vi "ReadWriteLoopCase3.vi"() -> ()   [LabVIEW 2019]
uses:
  <vilib>/DAQmx/read.llb/DAQmx Read (Analog DBL 1Chan 1Samp).vi
  <vilib>/DAQmx/write.llb/DAQmx Write (Analog DBL 1Chan 1Samp).vi
  <vilib>/DAQmx/create/channels.llb/DAQmx Create Channel (AI-Voltage-Basic).vi
  <vilib>/DAQmx/configure/timing.llb/DAQmx Timing (Sample Clock).vi
  <vilib>/DAQmx/create/channels.llb/DAQmx Create Channel (AO-Voltage-Basic).vi
  <vilib>/DAQmx/miscellaneous.llb/DAQmx Fill In Error Info.vi
  <resource>/objmgr/daqmx.rc
panel:
  out "error out":errorcluster
  out "Slide":dbl(slide) scale=2900.0..3100.0
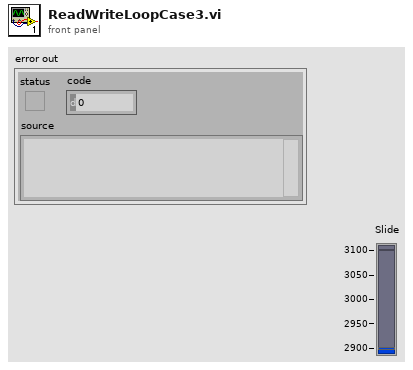
[diagram p1: front panel]
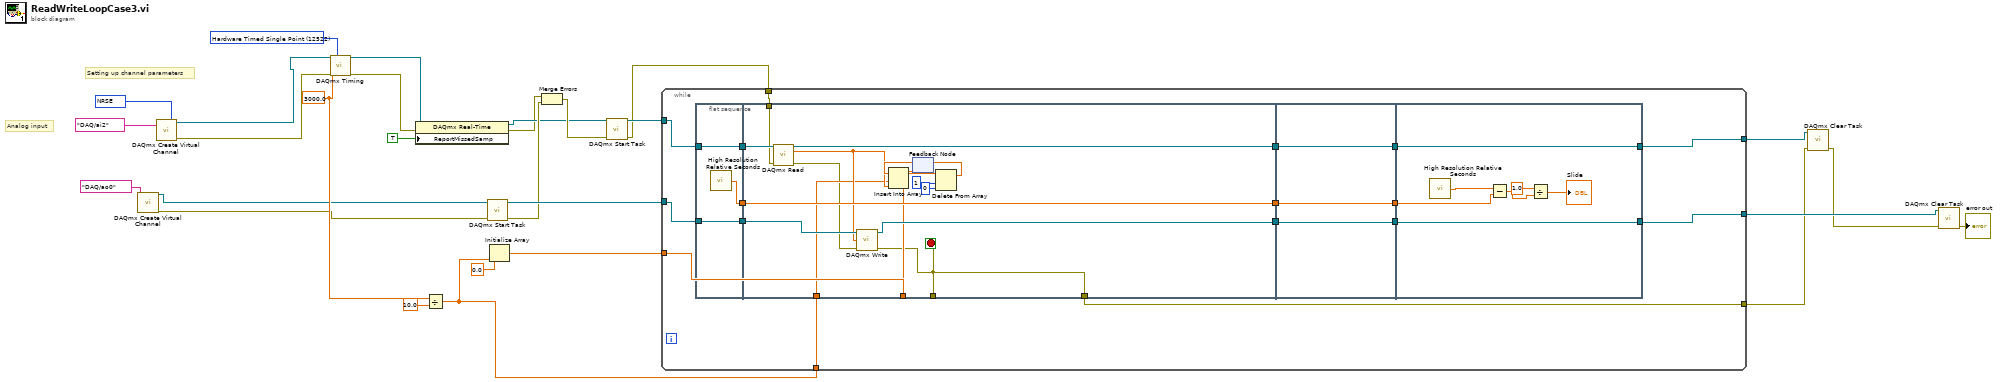
[diagram p0: block diagram]
diagram:
  w8 = 3000.0 ("rate")
  w23 = 12522 items=["Finite Samples"=10178, "Continuous Samples"=10123, "Hardware Timed Single Point"=12522] ("sample mode")
  w26 = 10078 items=["Default"=-1, "RSE"=10083, "NRSE"=10078, "Differential"=10106, "Pseudodifferential"=12529] ("input terminal configuration")
  # "Analog input"
  # "Setting up channel parameters"
  n1 = call-poly <vilib>:"DAQmx Create Virtual Channel.vi"("physical channels"=tag "DAQ/ao0") -> ("task out"=w2:refnum<k21>, "error out"=w1:errorcluster)  [unwired: 13 in]
  n2 = call-poly <vilib>:"DAQmx Create Virtual Channel.vi"("input terminal configuration"=w26, "physical channels"=tag "DAQ/ai2") -> ("task out"=w24:refnum<k21>, "error out"=w9:errorcluster)  [unwired: 12 in]
  n3 = call-poly <vilib>:"DAQmx Timing.vi"("task/channels in"=w24, "sample mode"=w23, "rate"=w8, "error in"=w9) -> ("task out"=w5:refnum<k21>, "error out"=w6:errorcluster)  [unwired: 10 in]
  n4 = property class="DAQmx Real-Time"(reference=w5, error in=w6, "ReportMissedSamp"=TRUE) -> (reference out=w4:refnum<k21>, error out=w3:errorcluster)
  n5 = Divide(x=w8, y=10.0) -> (x/y=w18:dbl)
  n6 = call <vilib>:"DAQmx Start Task.vi"("task/channels in"=w2, "error in"=w1) -> ("task out"=w27:refnum<k21>, "error out"=w17:errorcluster)  [unwired: 12 in]
  n7 = Initialize Array(0.0 ("element"), w18) -> (w21:dbl[])
  n8 = Merge Errors(w3, w17) -> (w16:errorcluster)
  n9 = call <vilib>:"DAQmx Start Task.vi"("task/channels in"=w4, "error in"=w16) -> ("task out"=w28:refnum<k21>, "error out"=w15:errorcluster)  [unwired: 12 in]
  n10 = while {
    tunnel: w28 -> [w45]
    tunnel: w27 -> [w44]
    tunnel: [w43] -> w14
    tunnel: [w42] -> w13
    tunnel: w21 -> [w32]
    tunnel: w18 -> [w31]
    tunnel: w15 -> [w30]
    tunnel: [w29] -> w12
    stop <- w46 stop-if-true
    n11 = flat-sequence {
      tunnel: w44 -> [w48]
      tunnel: w45 -> [w49]
      tunnel: [w49] -> w41
      tunnel: [w48] -> w40
      tunnel: [w47] -> w33
      tunnel: [w50] -> w46
      tunnel: w41 -> [w65]
      tunnel: w40 -> [w64]
      tunnel: [w63] -> w39
      tunnel: [w62] -> w38
      tunnel: [w61] -> w34
      tunnel: w33 -> [w61]
      tunnel: w32 -> [w57]
      tunnel: w31 -> [w53]
      tunnel: w30 -> [w52]
      tunnel: [w50] -> w29
      tunnel: w39 -> [w68]
      tunnel: w38 -> [w67]
      tunnel: [w68] -> w37
      tunnel: [w67] -> w36
      tunnel: [w66] -> w35
      tunnel: w34 -> [w66]
      tunnel: [w69] -> w42
      tunnel: [w75] -> w43
      tunnel: w37 -> [w75]
      tunnel: w36 -> [w69]
      tunnel: w35 -> [w73]
      frame #0 {
        n12 = call <vilib>:"High Resolution Relative Seconds.vi"() -> ("relative seconds"=w47:dbl)
      }
      frame #1 {
        n13 = call-poly <vilib>:"DAQmx Read.vi"("task/channels in"=w65, "error in"=w52) -> ("task out"=w63:refnum<k21>, "data"=w54:dbl, "error out"=w51:errorcluster)  [unwired: 11 in]
        n14 = call-poly <vilib>:"DAQmx Write.vi"("task/channels in"=w64, "data"=w54, "error in"=w51) -> ("task out"=w62:refnum<k21>, "error out"=w50:errorcluster)  [unwired: 10 in, 1 out]
        n15 = feedback #1(w57) -> (w60:dbl[])
        n16 = Insert Into Array(array=w60, index=w53, new element=w54) -> (w56:dbl[])
        n17 = Delete From Array(array=w56, length=1, index=0) -> (array with subset deleted=w55:dbl[])  [unwired: 1 out]
        n18 = feedback-in #1(w55) -> ()
      }
      frame #2 {
      }
      frame #3 {
        n19 = call <vilib>:"High Resolution Relative Seconds.vi"() -> ("relative seconds"=w74:dbl)
        n20 = Subtract(x=w74, y=w73) -> (x-y=w71:dbl)
        n21 = Divide(x=1.0, y=w71) -> (x/y=→"Slide":dbl)
      }
    }
  }
  n22 = call <vilib>:"DAQmx Clear Task.vi"("task in"=w14, "error in"=w12) -> ("error out"=w11:errorcluster)  [unwired: 13 in]
  n23 = call <vilib>:"DAQmx Clear Task.vi"("task in"=w13, "error in"=w11) -> ("error out"=→"error out":errorcluster)  [unwired: 13 in]
